vi "SetShutterStatus.vi"(8 "error in (no error)":errorcluster, 9 "Value":bool, 10 "Label":string, 11 "Laser_Oxxius in":refnum<class "Laser_Oxxius.lvclass">) -> (0 "error out":errorcluster, 3 "Laser_Oxxius out":refnum<class "Laser_Oxxius.lvclass">)   [LabVIEW 2020, in "Laser_Oxxius.lvlib" / "Laser_Oxxius.lvclass"]
uses:
  Laser_Oxxius.lvclass
  Laser_Oxxius.lvclass/Laser_Oxxius.ctl
  D:/Daguan/Development/MMicroscopyAF/Model/Hardware Layer/Real Hardware/Laser_Oxxius/Laser_Oxxius/Dependency/Oxxius_Boxx.dll
  Dependency/Oxxius_Boxx.dll
  Hardware Abstraction Layer/Component/Laser/Laser/Laser.lvclass
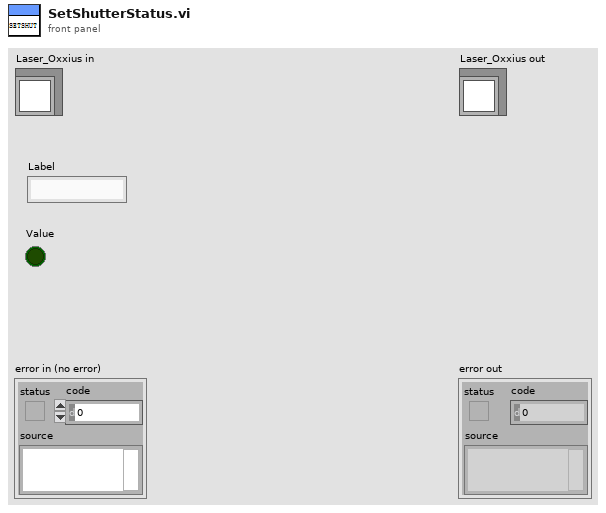
[diagram p1: front panel]
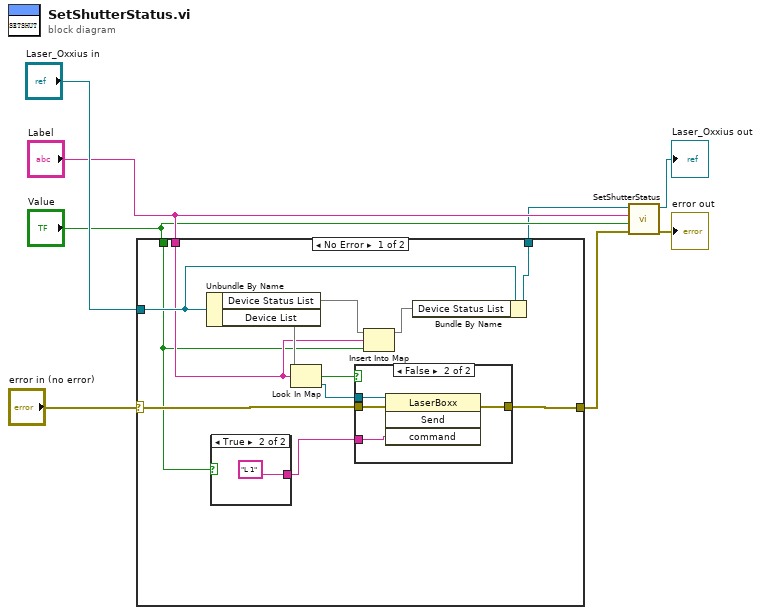
[diagram p0: block diagram]
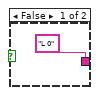
[diagram p2: hidden frame]
diagram:
  n1 = case shown="No Error" "error in (no error)" {
    selector: "error in (no error)" -> [w20 w29]
    tunnel: "Laser_Oxxius in" -> [w14 w28]
    tunnel: [w17 w29] -> w5
    tunnel: "Value" -> [w9 _]
    tunnel: "Label" -> [w10 _]
    tunnel: [w13 w28] -> w1
    frame No Error {
      n2 = Unbundle By Name(w14) -> ("Device Status List"=w12:map{string, bool}, "Device List"=w19:map{string, refnum<k24>})
      n3 = case shown="True" w9 {
        tunnel: ["L 0" ("command") "L 1" ("command")] -> w15
        frame False {
        }
        frame True {
        }
      }
      n4 = Look In Map(map=w19, key=w10) -> (key not found?=w16:bool, value=w18:refnum<k24>)  [unwired: 1 in]
      n5 = case shown="False" w16 {
        tunnel: w20 -> [w23 w27]
        tunnel: w18 -> [_ w26]
        tunnel: [w23 w25] -> w17
        tunnel: w15 -> [_ w24]
        frame True {
        }
        frame False {
          n6 = invoke class="LaserBoxx" method="Send"(reference=w26, error in=w27, "command"=w24) -> (error out=w25:errorcluster)  [unwired: 1 in, 3 out]
        }
      }
      n7 = Insert Into Map(map in=w12, key=w10, value=w9) -> (map out=w11:map{string, bool})  [unwired: 2 out]
      n8 = Bundle By Name(cluster=w14, "Device Status List"=w11) -> (w13:refnum<class "Laser_Oxxius.lvclass">)
    }
    frame Error {
    }
  }
  n9 = call-parent "SetShutterStatus.vi"("error in (no error)"=w5, "Value"="Value", "Label"="Label", "Laser in"=w1) -> ("error out"=→"error out":errorcluster, "Laser out"=→"Laser_Oxxius out":refnum<class "Laser_Oxxius.lvclass">)  [unwired: 6 in]
